vi "process.vi"(8 "error in (no error)":errorcluster, 11 "TCPConnectionHandler in":refnum<class "TCPConnectionHandler.lvclass">) -> (0 "error out":errorcluster, 3 "TCPConnectionHandler out":refnum<class "TCPConnectionHandler.lvclass">)   [LabVIEW 2013, in "MQTT_TCP.lvlib" / "TCPConnectionHandler.lvclass"]
uses:
  TCPConnectionHandler.lvclass
  TCPConnectionHandler.lvclass/TCPConnectionHandler.ctl
  Server/Session.Server/Session.Server.lvclass
  MQTT_Base/Session/Session.lvclass
  MQTT_Base/Session/Session.lvclass/Session.ctl
  <vilib>/Utility/error.llb/Clear Errors.vi
  Connection/TCPConnection.lvclass
  MQTT_Base/Base Class/MQTT_Base.lvclass
panel:
  out "Stored Connections":i32
  out "connection time (s)":dbl format="%.06f"
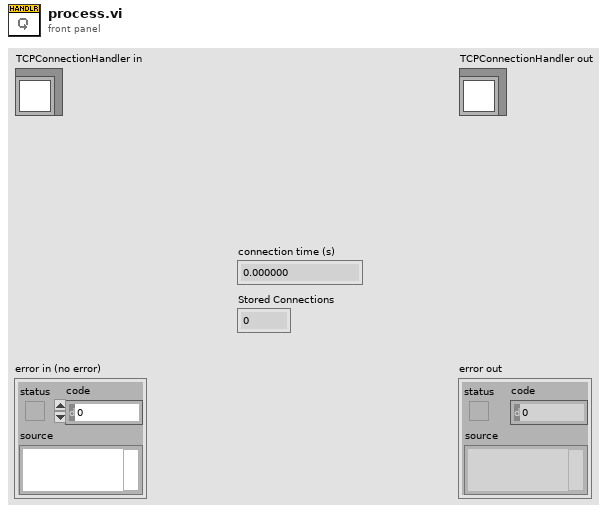
[diagram p1: front panel]
types:
  T1 = typedef "MQTT_TCP.lvlib/TCPConnectionHandler.lvclass/Private Events -- Cluster.ctl" = cluster{"Close Session Event":refnum<user-event>, "NbConnections":refnum<user-event>}
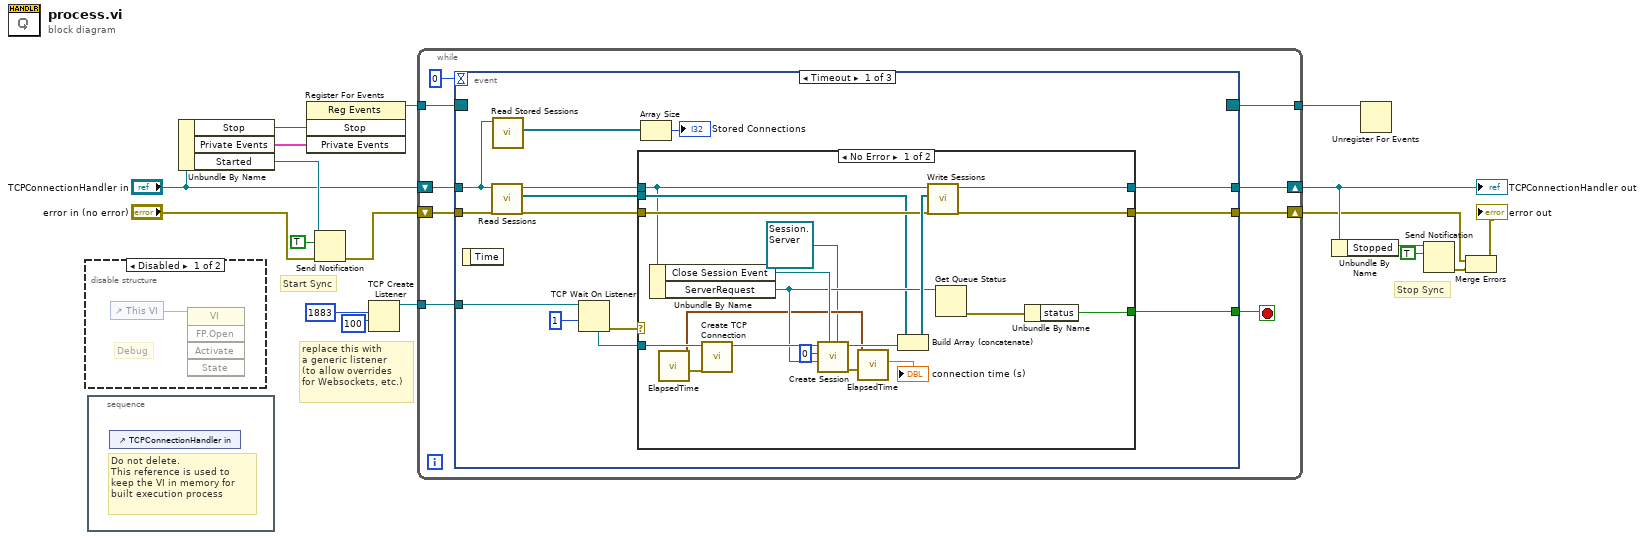
[diagram p0: block diagram]
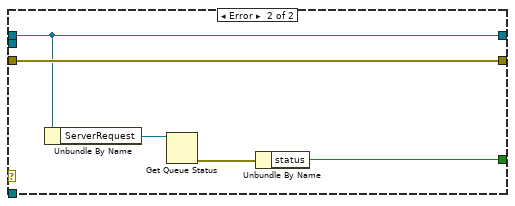
[diagram p3: hidden frame]
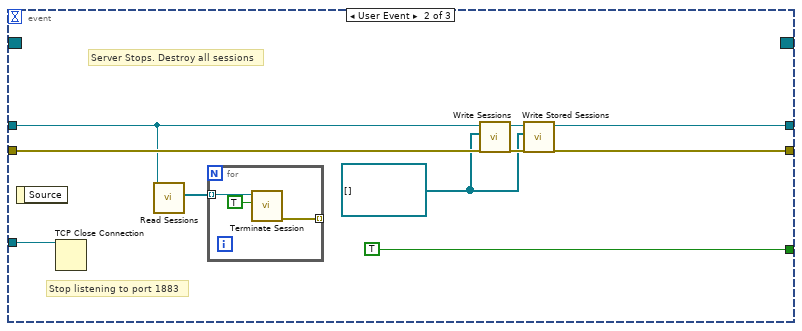
[diagram p4: hidden frame]
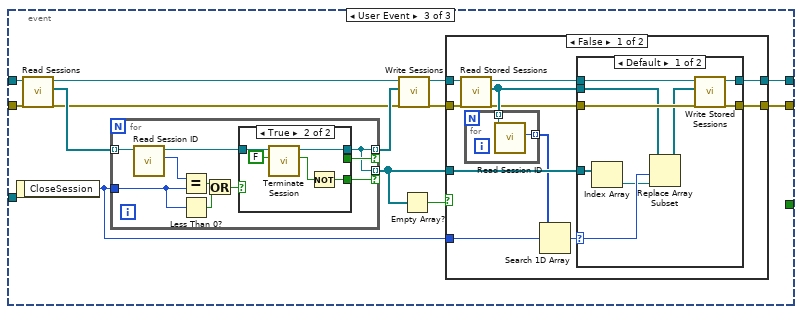
[diagram p5: hidden frame]
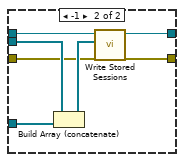
[diagram p6: hidden frame]
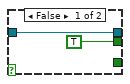
[diagram p8: hidden frame]
diagram:
  # "replace this with\na generic listener\n(to allow overrides\nfor Websockets, etc.)"
  # "Stop Sync"
  # "Start Sync"
  n1 = disable-structure shown="Disabled" {
    frame Disabled {
      # "Debug"
      n2 = control-ref of="This VI"() -> (w19:refnum<vi>)
      n3 = invoke class="VI" method="FP.Open"(reference=w19) -> ()  [unwired: 4 in, 5 out]
    }
    frame Enabled {
    }
  }
  n4 = stacked-sequence {
    frame #0 {
      # "Do not delete.\nThis reference is used to keep the VI in memory for built execution process"
      n5 = control-ref of="TCPConnectionHandler in"() -> ()  [unwired: 1 out]
    }
  }
  n6 = Unbundle By Name("TCPConnectionHandler in") -> ("Stop"=w18:refnum<user-event>, "Private Events"=w12:T1, "Started"=w9:refnum<notifier>)
  n7 = register-events(w18, w12) -> (reference out=w13:refnum<event-registration>)  [unwired: 2 in, 1 out]
  n8 = Send Notification(notification=TRUE, notifier=w9, error in (no error)="error in (no error)") -> (error out=w10:errorcluster)  [unwired: 1 out]
  n9 = TCP Create Listener(9:100, 10:u16 1883 ("port")) -> (3:w16:refnum<k5>)  [unwired: 3 in, 2 out]
  n10 = while {
    shift-right: [w25] -> w8
    shift-left: "TCPConnectionHandler in" -> [w24]
    shift-right: [w27] -> w3
    shift-left: w10 -> [w26]
    tunnel: w13 -> [w23]
    tunnel: [w22] -> w17
    tunnel: w16 -> [w20]
    stop <- w21 stop-if-true
    n11 = event shown="[0] Timeout" {
      selector: w23 -> [_ _ _]
      dyn-events: [_ _ _] -> w22
      timeout: 0 -> [_ _ _]
      tunnel: [w35 w72 w78] -> w27
      tunnel: w26 -> [w37 w72 w77]
      tunnel: [w36 w66 w84] -> w25
      tunnel: w24 -> [w31 w69 w82]
      tunnel: [w34 TRUE _] -> w21
      tunnel: w20 -> [w41 w68 _]
      event Timeout {
        n12 = event-data() -> ()  [unwired: 1 in, 1 out]
        n13 = call "Read Sessions.vi"("TCPConnectionHandler in"=w31) -> ("Sessions"=w32:refnum<class "Session.lvclass">[], "TCPConnectionHandler out"=w33:refnum<class "TCPConnectionHandler.lvclass">)  [unwired: 9 in]
        n14 = call "Read Stored Sessions.vi"("TCPConnectionHandler in"=w31) -> ("Stored Sessions"=w29:refnum<class "Session.lvclass">[])  [unwired: 9 in, 1 out]
        n15 = TCP Wait On Listener(9:1, 11:w41) -> (0:w39:errorcluster, 4:w38:refnum<k5>)  [unwired: 2 in, 3 out]
        n16 = case shown="No Error" w39 {
          tunnel: w38 -> [w59 _]
          tunnel: w33 -> [w47 w63]
          tunnel: w37 -> [w54 w64]
          tunnel: [w53 w63] -> w36
          tunnel: [w54 w64] -> w35
          tunnel: [w49 w60] -> w34
          tunnel: w32 -> [w48 _]
          frame No Error {
            n17 = Unbundle By Name(w47) -> ("Close Session Event"=w52:refnum<user-event>, "ServerRequest"=w50:refnum<queue>)
            n18 = call "ElapsedTime.vi"() -> ("error out"=w46:errorcluster, "current time"=w44:timestamp)  [unwired: 9 in, 1 out]
            n19 = call "Create TCP Connection.vi"("error in (no error)"=w46, "connection ID"=w59) -> ("TCPConnection out"=w58:refnum<class "TCPConnection.lvclass">)  [unwired: 8 in, 1 out]
            n20 = call "Create Session.vi"("Session in"=refnum<class "Session.Server.lvclass"> refnum ("MQTT Server.lvlib:Session.Server.lvclass"), "Close Session"=w52, "Request"=w50, "Keep Alive (s)"=0, "Connection"=w58) -> ("error out"=w45:errorcluster, "Session"=w56:refnum<class "Session.Server.lvclass">)  [unwired: 5 in]
            n21 = call "ElapsedTime.vi"("error in"=w45, "compare time"=w44) -> ("elapsed (s)"=→"connection time (s)":dbl)  [unwired: 7 in, 2 out]
            n22 = Build Array (concatenate)(w48, w56) -> (w55:refnum<class "Session.lvclass">[])
            n23 = call "Write Sessions.vi"("Sessions"=w55, "TCPConnectionHandler in"=w47) -> ("TCPConnectionHandler out"=w53:refnum<class "TCPConnectionHandler.lvclass">)  [unwired: 9 in]
            n24 = Get Queue Status(queue=w50) -> (error out=w51:errorcluster)  [unwired: 2 in, 7 out]
            n25 = Unbundle By Name(w51) -> ("status"=w49:bool)
          }
          frame Error {
            n26 = Unbundle By Name(w63) -> ("ServerRequest"=w62:refnum<queue>)
            n27 = Get Queue Status(queue=w62) -> (error out=w61:errorcluster)  [unwired: 2 in, 7 out]
            n28 = Unbundle By Name(w61) -> ("status"=w60:bool)
          }
        }
        n29 = Array Size(array=w29) -> (size(s)=→"Stored Connections":i32)
      }
      event User Event {
        w65 = refnum<class "Session.lvclass">[] [] ("Sessions")
        # "Stop listening to port 1883"
        # "Server Stops. Destroy all sessions"
        n30 = event-data() -> ()  [unwired: 1 in, 1 out]
        n31 = TCP Close Connection(connection ID=w68) -> ()  [unwired: 2 in, 2 out]
        n32 = call "Read Sessions.vi"("TCPConnectionHandler in"=w69) -> ("Sessions"=w70:refnum<class "Session.lvclass">[])  [unwired: 9 in, 1 out]
        n33 = for {
          tunnel: w70 -> [w75] mode=indexing
          tunnel: [w74] -> _ mode=indexing
          n34 = call "Terminate Session.vi"("Destroy (T)"=TRUE, "Session in"=w75) -> ("error out"=w74:errorcluster)  [unwired: 7 in, 2 out]
        }
        n35 = call "Write Sessions.vi"("Sessions"=w65, "TCPConnectionHandler in"=w69) -> ("TCPConnectionHandler out"=w67:refnum<class "TCPConnectionHandler.lvclass">)  [unwired: 9 in]
        n36 = call "Write Stored Sessions.vi"("Stored Sessions"=w65, "TCPConnectionHandler in"=w67) -> ("TCPConnectionHandler out"=w66:refnum<class "TCPConnectionHandler.lvclass">)  [unwired: 9 in]
      }
      event User Event {
        n37 = event-data() -> ("CloseSession"=w76:i32)  [unwired: 1 in]
        n38 = call "Read Sessions.vi"("TCPConnectionHandler in"=w82) -> ("Sessions"=w86:refnum<class "Session.lvclass">[], "TCPConnectionHandler out"=w81:refnum<class "TCPConnectionHandler.lvclass">)  [unwired: 9 in]
        n39 = for {
          tunnel: w86 -> [w123] mode=indexing
          tunnel: [w116] -> w85 mode=indexing if=w124
          tunnel: w76 -> [w118]
          tunnel: [w116] -> w80 mode=indexing if=w115
          n40 = call "Read Session ID.vi"("Session in"=w123) -> ("Session ID"=w121:i32, "Session out"=w122:refnum<class "Session.lvclass">)  [unwired: 8 in, 1 out]
          n41 = Equal?(x=w121, y=w118) -> (x = y?=w120:bool)
          n42 = Less Than 0?(x=w118) -> (x < 0?=w119:bool)
          n43 = Or(x=w120, y=w119) -> (x .or. y?=w117:bool)
          n44 = case shown="True" w117 {
            tunnel: w122 -> [w126 w131]
            tunnel: [w126 w130] -> w116
            tunnel: [TRUE _] -> w124
            tunnel: [_ w127] -> w115
            frame False {
            }
            frame True {
              n45 = call "Terminate Session.vi"("Destroy (T)"=FALSE, "Session in"=w131) -> ("Destroyed"=w128:bool, "Session out"=w130:refnum<class "Session.lvclass">)  [unwired: 7 in, 1 out]
              n46 = Not(x=w128) -> (.not. x?=w127:bool)
            }
          }
        }
        n47 = call "Write Sessions.vi"("Sessions"=w85, "TCPConnectionHandler in"=w81) -> ("TCPConnectionHandler out"=w83:refnum<class "TCPConnectionHandler.lvclass">)  [unwired: 9 in]
        n48 = Empty Array?(array=w80) -> (empty?=w79:bool)
        n49 = case shown="False" w79 {
          tunnel: [w96 w114] -> w84
          tunnel: w83 -> [w95 w114]
          tunnel: w80 -> [w93 _]
          tunnel: [w87 w113] -> w78
          tunnel: w77 -> [w88 w113]
          tunnel: w76 -> [w90 _]
          frame False {
            n50 = call "Read Stored Sessions.vi"("TCPConnectionHandler in"=w95) -> ("Stored Sessions"=w92:refnum<class "Session.lvclass">[], "TCPConnectionHandler out"=w94:refnum<class "TCPConnectionHandler.lvclass">)  [unwired: 9 in]
            n51 = for {
              tunnel: w92 -> [w112] mode=indexing
              tunnel: [w111] -> w91 mode=indexing
              n52 = call "Read Session ID.vi"("Session in"=w112) -> ("Session ID"=w111:i32)  [unwired: 8 in, 2 out]
            }
            n53 = Search 1D Array(1D array=w91, element=w90) -> (index of element=w89:i32)  [unwired: 1 in]
            n54 = case shown="Default" w89 {
              selector: w89 -> [w100 _]
              tunnel: [w104 w110] -> w96
              tunnel: w94 -> [w102 w109]
              tunnel: w93 -> [w99 w107]
              tunnel: w92 -> [w101 w106]
              tunnel: w88 -> [w103 w105]
              tunnel: [w103 w105] -> w87
              frame Default {
                n55 = Index Array(array=w99) -> (element=w98:refnum<class "Session.lvclass">)  [unwired: 1 in]
                n56 = Replace Array Subset(array=w101, new element=w98, index=w100) -> (w97:refnum<class "Session.lvclass">[])
                n57 = call "Write Stored Sessions.vi"("Stored Sessions"=w97, "TCPConnectionHandler in"=w102) -> ("TCPConnectionHandler out"=w104:refnum<class "TCPConnectionHandler.lvclass">)  [unwired: 9 in]
              }
              frame -1 {
                n58 = Build Array (concatenate)(w106, w107) -> (w108:refnum<class "Session.lvclass">[])
                n59 = call "Write Stored Sessions.vi"("Stored Sessions"=w108, "TCPConnectionHandler in"=w109) -> ("TCPConnectionHandler out"=w110:refnum<class "TCPConnectionHandler.lvclass">)  [unwired: 9 in]
              }
            }
          }
          frame True {
          }
        }
      }
    }
  }
  "TCPConnectionHandler out" <- w8
  n60 = Unbundle By Name(w8) -> ("Stopped"=w7:refnum<notifier>)
  n61 = Unregister For Events(event registration refnum=w17) -> ()  [unwired: 1 in, 1 out]
  n62 = Send Notification(notification=TRUE, notifier=w7) -> (error out=w4:errorcluster)  [unwired: 1 in, 1 out]
  n63 = Merge Errors(w3, w4) -> (→"error out":errorcluster)
